vi "GWInstek  GDM8351 Acquire Single.vi"() -> ()   [LabVIEW 2021]
doc: "This example shows how to configure a measurement and take a reading."
uses:
  <instrlib>/GWInstek  GDM8351/Public/Data/Read (Single Point).vi
  <instrlib>/GWInstek  GDM8351/GWInstek  GDM8351.lvlib
panel:
  in  "Function (0: DC Volts)":i32(ring) items=["DC Volts", "AC Volts", "DC+AC Volts", "DC Current", "AC Current", "DC+AC Current", "2-Wire Resistance", "4-Wire Resistance", "Frequency", "Period", "Continuity", "Diode", "Temperature", "Capacitance"]
  in  "Baud Rate (115200)":u32(ring)=115200 items=["9600"=9600, "19200"=19200, "38400"=38400, "57600"=57600, "115200"=115200]
  in  "Rate (0: Slow)":i32(ring) items=["Slow", "Mid", "Fast"]
  in  "Range (1.0)":dbl=1.0
  out "Measurement":dbl
  in  "VISA resource name":refnum<visa-resource-name>
  # "(c) 2014 GWInstek.  ALL RIGHTS RESERVED."
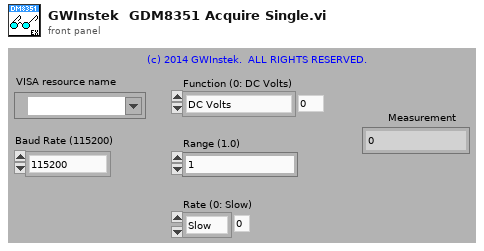
[diagram p1: front panel]
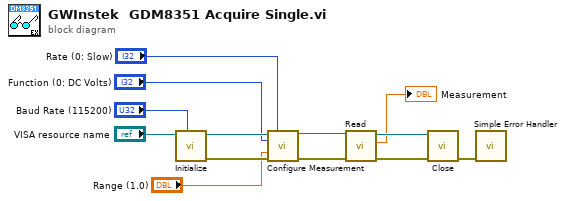
[diagram p0: block diagram]
diagram:
  n1 = call <instrlib>:"Initialize.vi"("Baud Rate (115200)"="Baud Rate (115200)", "VISA resource name"="VISA resource name") -> ("error out"=w10:errorcluster, "VISA resource name out"=w11:refnum<visa-resource-name>)  [unwired: 8 in]
  n2 = call <instrlib>:"Configure Measurement.vi"("VISA resource name"=w11, "Rate (0: Slow)"="Rate (0: Slow)", "Function (0: DC Volts)"="Function (0: DC Volts)", "Manual Range (1.0)"="Range (1.0)", "error in (no error)"=w10) -> ("VISA resource name out"=w7:refnum<visa-resource-name>, "error out"=w6:errorcluster)  [unwired: 9 in]
  n3 = call-poly <instrlib>:"Read.vi"("error in (no error)"=w6, "VISA resource name"=w7) -> ("error out"=w9:errorcluster, "Measurement"=→"Measurement":dbl, "VISA resource name out"=w8:refnum<visa-resource-name>)  [unwired: 7 in]
  n4 = call <instrlib>:"Close.vi"("error in (no error)"=w9, "VISA resource name"=w8) -> ("error out"=w13:errorcluster)  [unwired: 9 in]
  n5 = call <vilib>:"Simple Error Handler.vi"("error in (no error)"=w13) -> ()  [unwired: 4 in, 5 out]
